vi "path_empty_check.vi"(8 "error in":errorcluster, 11 "path_Input":path) -> (0 "error out":errorcluster, 2 "bo_exist":bool, 3 "bo_Empty":bool)   [LabVIEW 2026]
doc: "this subVI checks if the path is emptyi"
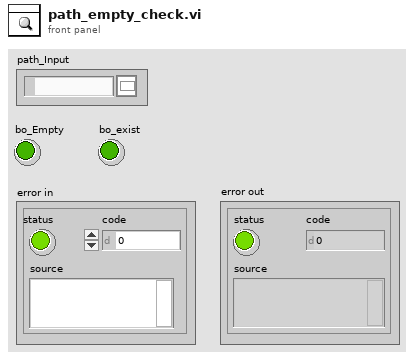
[diagram p1: front panel]
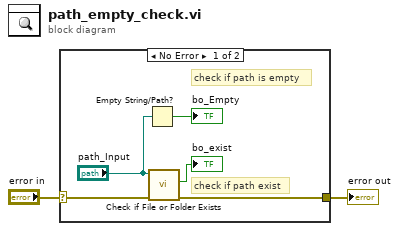
[diagram p0: block diagram]
diagram:
  n1 = case shown="No Error" "error in" {
    selector: "error in" -> [w3 w8]
    tunnel: [w5 w8] -> w2
    frame No Error {
      # "check if path exist"
      # "check if path is empty"
      n2 = Empty String/Path?(string/path="path_Input") -> (empty?=→"bo_Empty":bool)
      n3 = call <vilib>:"Check if File or Folder Exists.vi"("error in (no error)"=w3, "path"="path_Input") -> ("error out"=w5:errorcluster, "file or folder exists?"=→"bo_exist":bool)  [unwired: 7 in, 1 out]
    }
    frame Error {
    }
  }
  "error out" <- w2
